vi "Ini_file_RW_StrArrGen.vi"(4 "Section":string="Init", 5 "Key":string="Key1", 6 "FileName":string="Config", 7 "Error in":errorcluster, 8 "FolderSource":T1(ring)=enum."Répertoire du parent 1" caption="SaveFolderSource", 9 "Write":bool, 10 "ValueIn":string[](array[string])) -> (0 "Error out":errorcluster, 1 "file path":path caption="chemin du fichier", 3 "ValueOut":string[](array[string]))   [LabVIEW 2019]
doc: "Ce VI ouvre le fichier de sauvegarde des modèles et lit les positions du modèle spécifié."
uses:
  <vilib>/Utility/config.llb/Read Key (String).vi
  <vilib>/Utility/config.llb/Write Key (String).vi
  <vilib>/Utility/config.llb/NI_LVConfig.lvlib
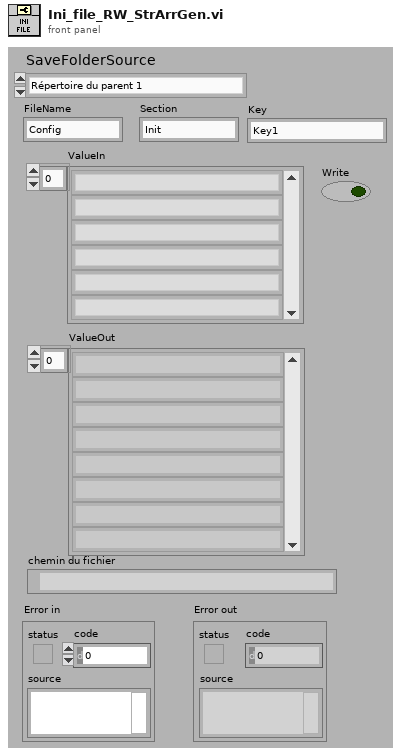
[diagram p1: front panel]
types:
  T1 = enum16{"Répertoire du VI actuel", "Répertoire du parent 1", "Répertoire du parent 2", "Répertoire du parent 3"}
  T2 = typedef "NI_LVConfig.lvlib/Config Data RefNum.ctl" = refnum<k1>
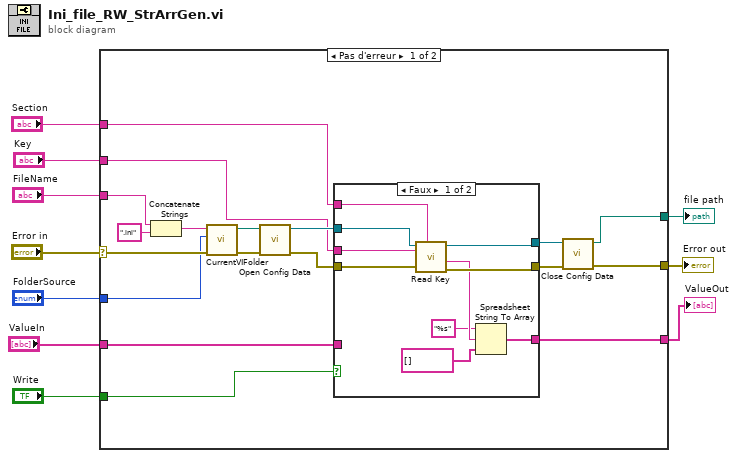
[diagram p0: block diagram]
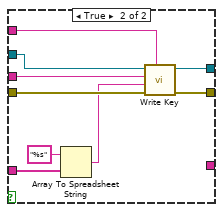
[diagram p2: hidden frame]
diagram:
  n1 = case shown="Pas d'erreur" "Error in" {
    selector: "Error in" -> [w23 w48]
    tunnel: [w22 w48] -> w10
    tunnel: "ValueIn" -> [w20 _]
    tunnel: "Write" -> [w19 _]
    tunnel: [w18 _] -> w6
    tunnel: "FileName" -> [w17 _]
    tunnel: "Key" -> [w14 _]
    tunnel: "Section" -> [w13 _]
    tunnel: "FolderSource" -> [w12 _]
    tunnel: [w11 _] -> w1
    frame No Error {
      n2 = Concatenate Strings(w17, ".ini" ("chaîne")) -> (w16:string)
      n3 = call <userlib>:"CurrentVIFolder.vi"("error in (no error)"=w23, "Source"=w12, "NomFichier"=w16) -> ("error out"=w28:errorcluster, "Chemin"=w21:path)  [unwired: 6 in, 1 out]
      n4 = call <vilib>:"Open Config Data.vi"("error in (no error)"=w28, "configuration file path"=w21) -> ("error out"=w25:errorcluster, "refnum"=w27:T2)  [unwired: 7 in, 1 out]
      n5 = case shown="Faux" w19 {
        tunnel: w27 -> [w35 w40]
        tunnel: w13 -> [w37 w47]
        tunnel: [w34 w46] -> w26
        tunnel: w25 -> [w38 w45]
        tunnel: [w33 w44] -> w24
        tunnel: w20 -> [_ w41]
        tunnel: w14 -> [w36 w39]
        tunnel: [w29 _] -> w18
        frame False {
          n6 = call-poly <vilib>:"Read Key.vi"("section"=w37, "error in (no error)"=w38, "key"=w36, "refnum"=w35) -> ("error out"=w33:errorcluster, "value"=w32:string, "refnum out"=w34:T2)  [unwired: 4 in, 1 out]
          n7 = Spreadsheet String To Array(format string="%s" ("chaîne de format"), spreadsheet string=w32, array type (2D Dbl)=string[] [] ("Filter names in")) -> (array=w29:string[])  [unwired: 1 in]
        }
        frame True {
          n8 = Array To Spreadsheet String(array=w41, 3:"%s" ("chaîne de format")) -> (spreadsheet string=w42:string)  [unwired: 1 in]
          n9 = call-poly <vilib>:"Write Key.vi"("section"=w47, "error in (no error)"=w45, "value"=w42, "key"=w39, "refnum"=w40) -> ("error out"=w44:errorcluster, "refnum out"=w46:T2)  [unwired: 4 in, 1 out]
        }
      }
      n10 = call <vilib>:"Close Config Data.vi"("error in (no error)"=w24, "refnum"=w26) -> ("error out"=w22:errorcluster, "file path"=w11:path)  [unwired: 8 in]
    }
    frame Error {
    }
  }
  "Error out" <- w10
  "ValueOut" <- w6
  "file path" <- w1
